vi "StopClone.vi"(8 "error in (no error)":errorcluster, 9 "Wait for Module to stop?":bool, 11 "ModuleAdmin":refnum<class "ModuleAdmin.lvclass">) -> (0 "error out":errorcluster)   [LabVIEW 2018, in "AcPwrShared.lvlib"]
doc: "This VI sends a message to Main.vi indicating it should stop its current activity and close."
uses:
  AcPwrShared/AcPwrShared.lvlib
  <userlib>/NIST/ModuleAdminLib/ModuleAdmin/ModuleAdmin.lvclass
  AcPwrModule.lvlib
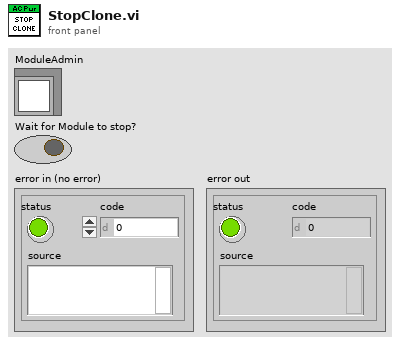
[diagram p1: front panel]
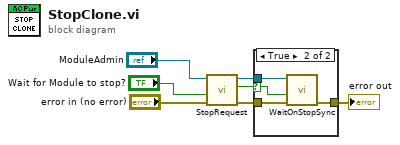
[diagram p0: block diagram]
diagram:
  n1 = call "StopRequest.vi"("error in (no error)"="error in (no error)", "Wait for Module to stop? (F)"="Wait for Module to stop?", "ModuleAdminIn"="ModuleAdmin") -> ("error out"=w3:errorcluster, "Wait to Stop"=w4:bool, "ModuleAdminOut"=w1:refnum<class "ModuleAdmin.lvclass">)  [unwired: 6 in]
  n2 = case shown="True" w4 {
    selector: w4 -> [_ w9]
    tunnel: [w8 w12] -> w7
    tunnel: w3 -> [w8 w11]
    tunnel: w1 -> [_ w10]
    frame False {
    }
    frame True {
      n3 = call <userlib>:"WaitOnStopSync.vi"("error in (no error)"=w11, "WaitForModuleToStop?"=w9, "ModuleAdmin"=w10) -> ("error out"=w12:errorcluster)  [unwired: 7 in, 1 out]
    }
  }
  "error out" <- w7
